vi "loop-iteration-terminal-visibility.vi"   [LabVIEW 2025]
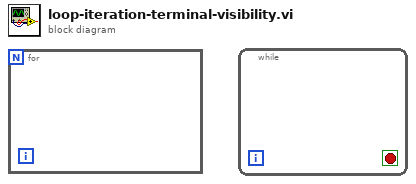
[diagram p0: block diagram]
diagram:
  n1 = for {
  }
  n2 = while {
    stop <- _ stop-if-true
  }
